vi "End.vi"(8 "error in (no error)":errorcluster, 11 "Client in":refnum<class "Client.lvclass">) -> (0 "error out":errorcluster, 3 "Client out":refnum<class "Client.lvclass">)   [LabVIEW 2018, in "Client.lvclass"]
uses:
  Client.lvclass
  Comm/Stream/Stream.lvclass
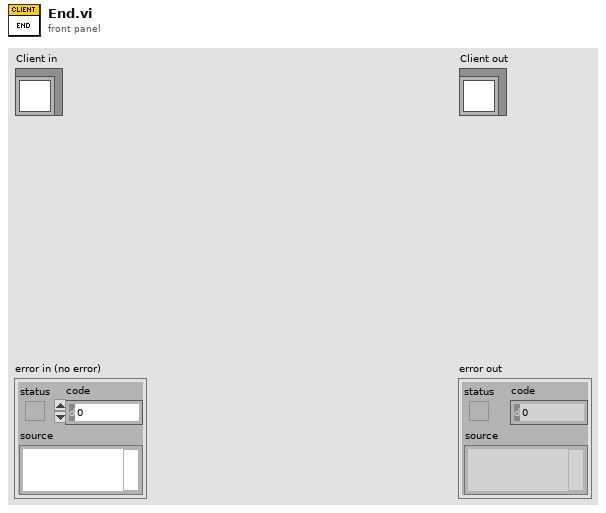
[diagram p1: front panel]
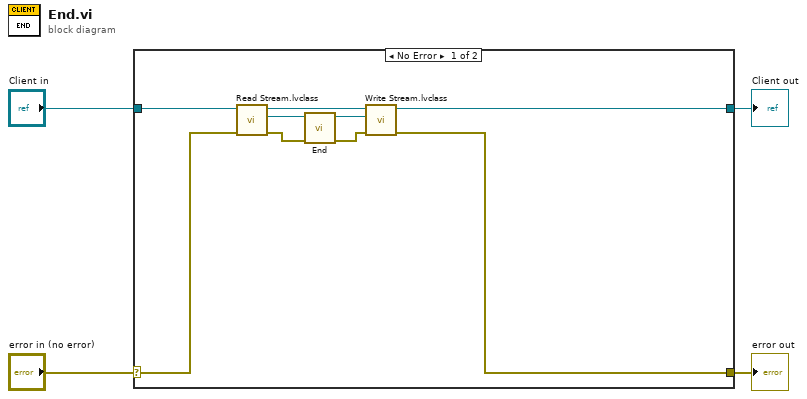
[diagram p0: block diagram]
diagram:
  n1 = case shown="No Error" "error in (no error)" {
    selector: "error in (no error)" -> [w7 w15]
    tunnel: [w5 w15] -> w3
    tunnel: [w6 w14] -> w1
    tunnel: "Client in" -> [w8 w14]
    frame No Error {
      n2 = call-dynamic "Read Stream.lvclass.vi"("error in (no error)"=w7, "Client in"=w8) -> ("error out"=w12:errorcluster, "Stream.lvclass"=w13:refnum<class "Stream.lvclass">, "Client out"=w9:refnum<class "Client.lvclass">)  [unwired: 7 in]
      n3 = call-dynamic "End.vi"("error in (no error)"=w12, "Stream in"=w13) -> ("error out"=w10:errorcluster, "Stream out"=w11:refnum<class "Stream.lvclass">)  [unwired: 8 in]
      n4 = call-dynamic "Write Stream.lvclass.vi"("error in (no error)"=w10, "Stream.lvclass"=w11, "Client in"=w9) -> ("error out"=w5:errorcluster, "Client out"=w6:refnum<class "Client.lvclass">)  [unwired: 7 in]
    }
    frame Error {
    }
  }
  "error out" <- w3
  "Client out" <- w1
